vi "History.vi"() -> ()   [LabVIEW 2019]
uses:
  <vilib>/httpClient/LabVIEWHTTPClient.lvlib
  <vilib>/NI/AMC/AMC.lvlib
  <vilib>/addons/_JKI.lib/Serialization/JSON/JKI JSON Serialization.lvlib
  <vilib>/NI/Tools/String/Tools_String.lvlib
  <vilib>/Utility/miscctls.llb/LVPointTypeDef.ctl
  SCADA/Archive Viewer/TraceData.ctl
panel:
  in  "Data is log (value)":bool
  in  "seconds between data points (1 to 300 sec)":i32=10 min=1 max=300 step=1
  out "Calls to server":i32
  out "Num Points Returned":i32
  in  "Log Scale":bool
  out "XY Graph":cluster{timestamp[], dbl[]}[](graph)
  in  "Plot Data":bool
  in  "End Time":timestamp
  in  "Start Time":timestamp
  in  "Exit":bool
  in  "Select Traces":i32[](listbox)
  in  "Select Database":i32(listbox)
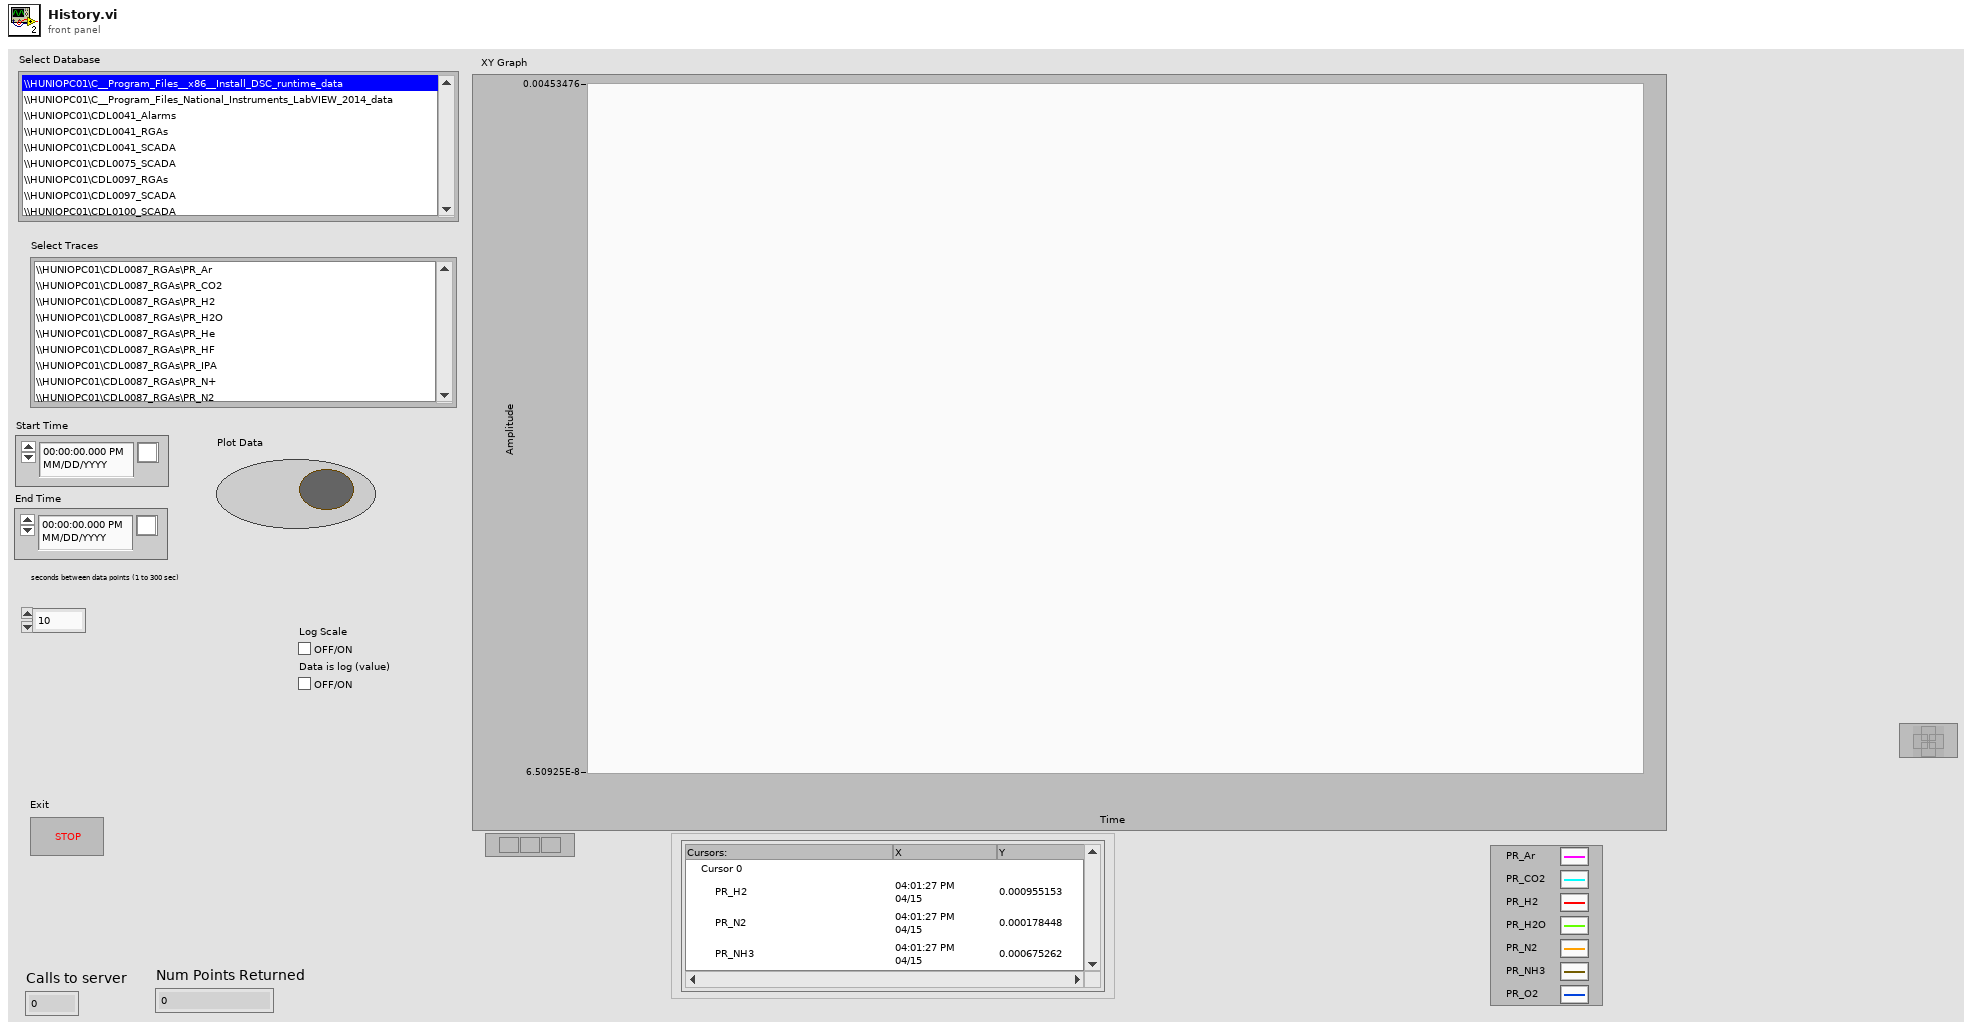
[diagram p1: front panel]
types:
  T1 = typedef "AMC.lvlib/Message Queue.ctl" = refnum<queue>
  T2 = typedef "LabVIEWHTTPClient.lvlib/ClientHandle.ctl" = refnum<k1>
  T3 = cluster{"firstTimestamp":string, "sampleInterval":i32, "data":dbl[]}
  T4 = typedef "LVPointTypeDef.ctl" = cluster{"Horizontal":i16, "Vertical":i16}
  T5 = typedef "TraceData.ctl" = cluster{"Trace":string, "LineWidth":u8, "TraceColor":u32, "DisplayName":string}
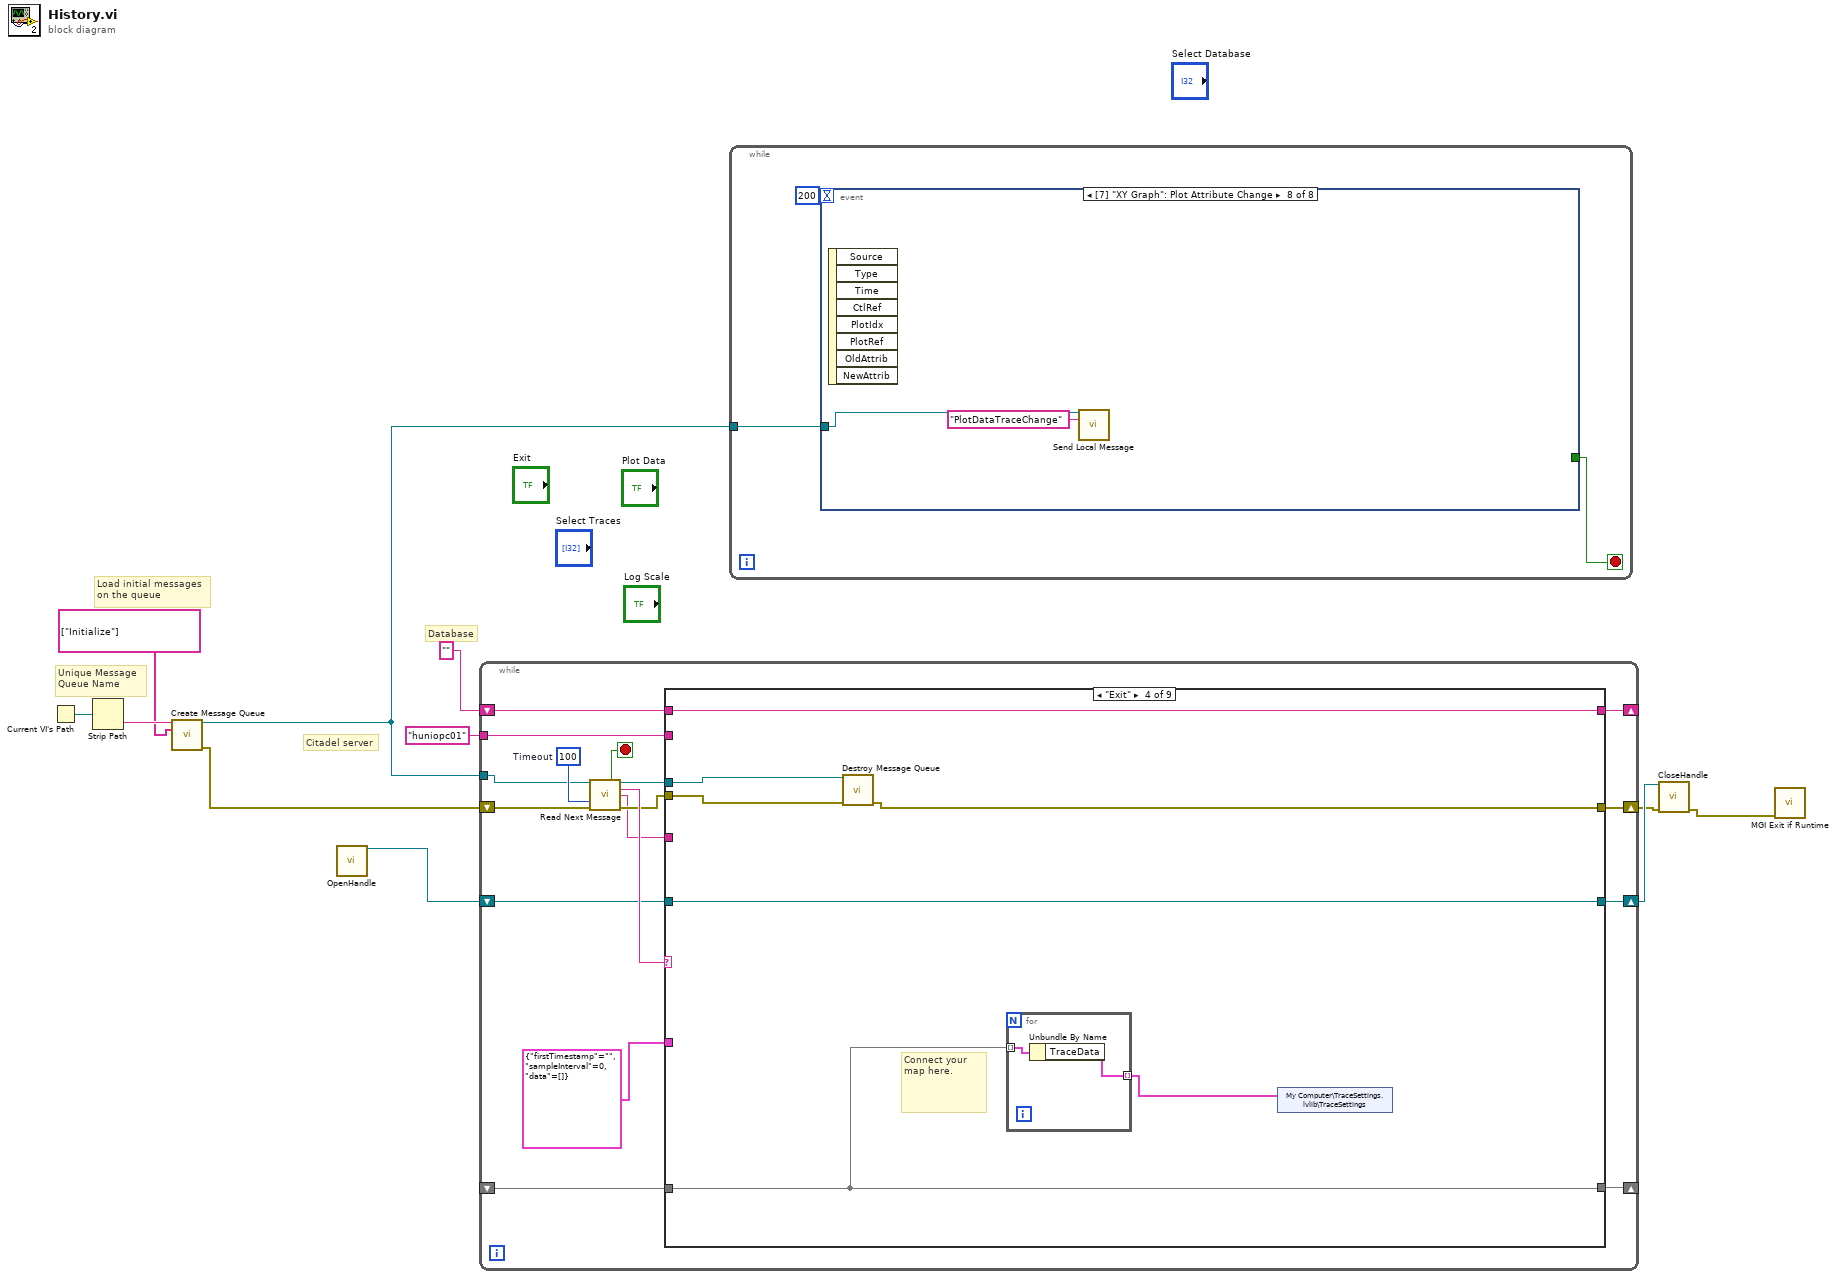
[diagram p0: block diagram]
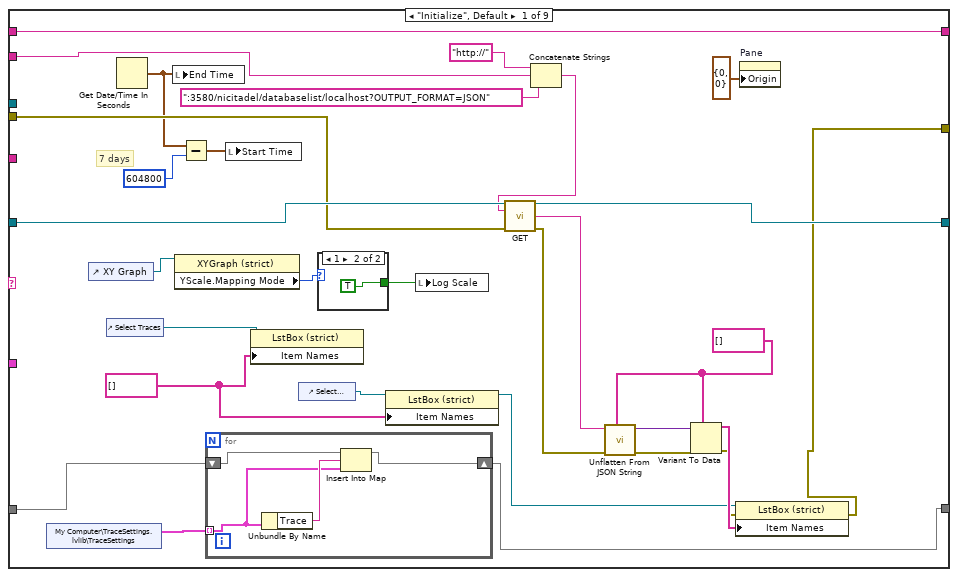
[diagram p2: hidden frame]
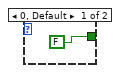
[diagram p3: hidden frame]
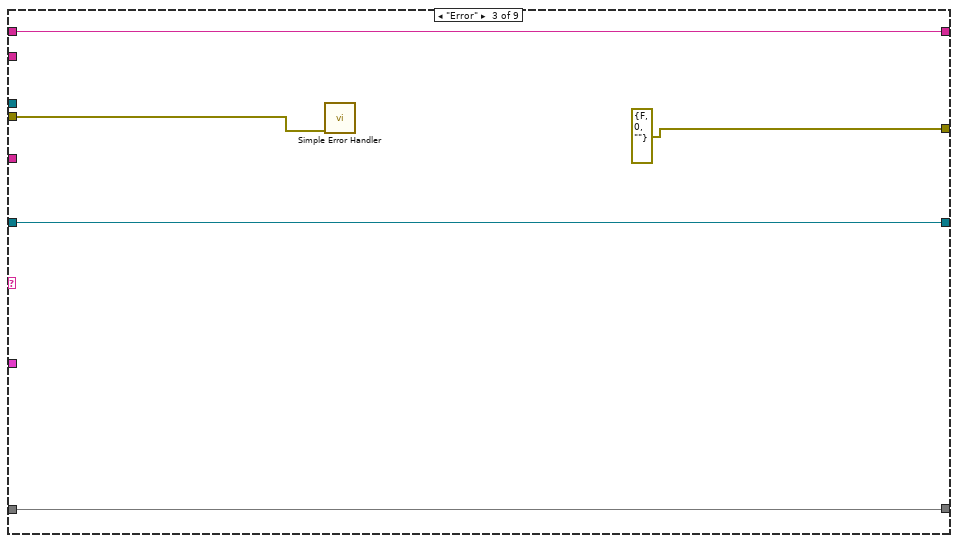
[diagram p5: hidden frame]
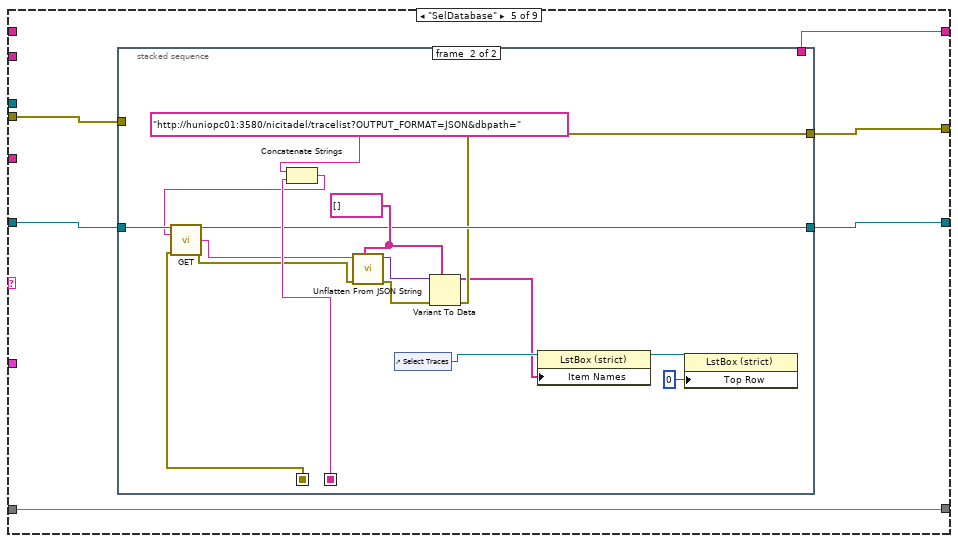
[diagram p6: hidden frame]
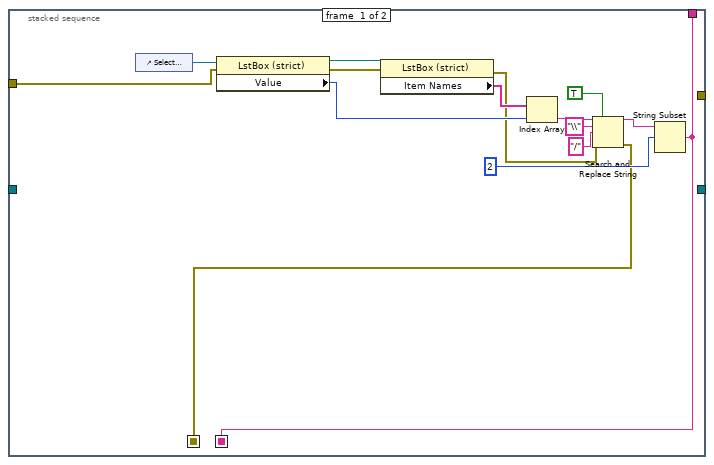
[diagram p7: hidden frame]
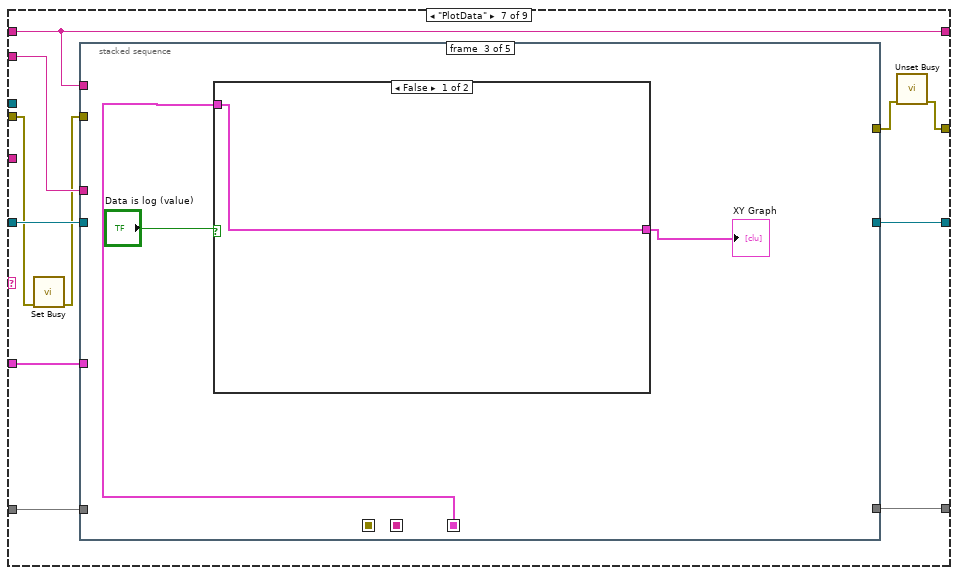
[diagram p9: hidden frame]
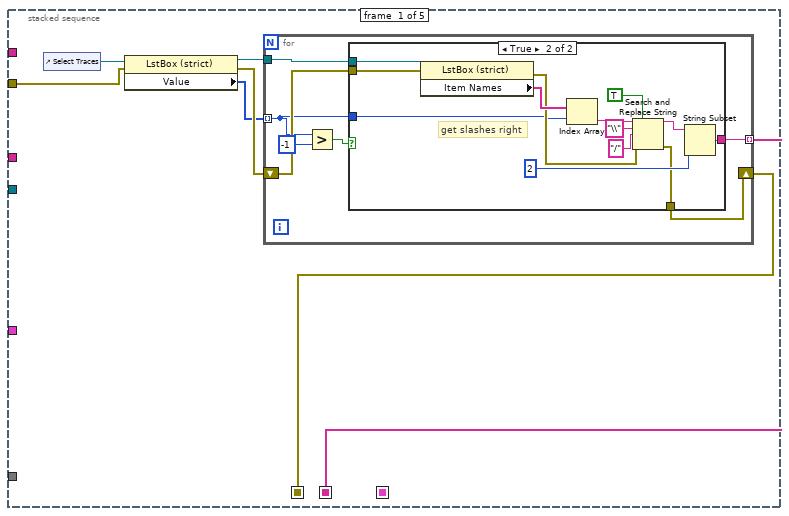
[diagram p10: hidden frame]
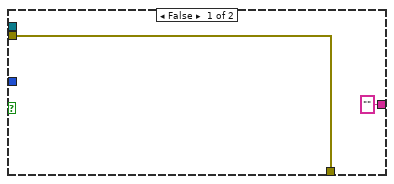
[diagram p11: hidden frame]
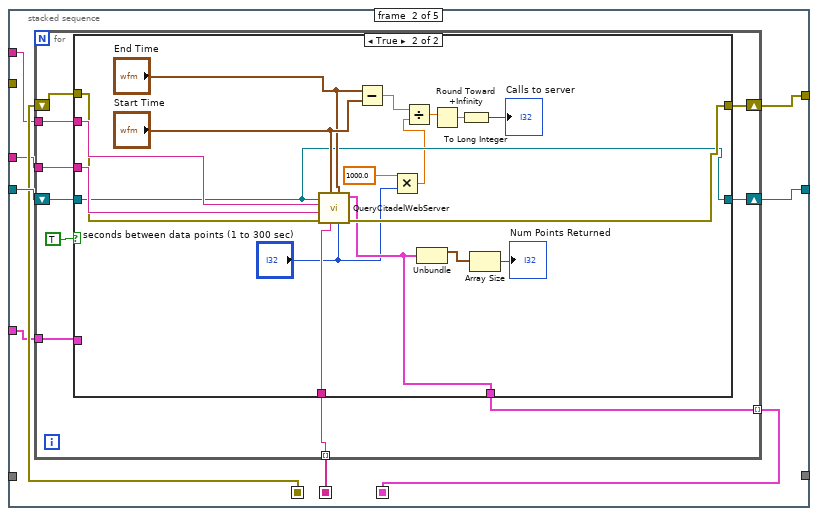
[diagram p12: hidden frame]
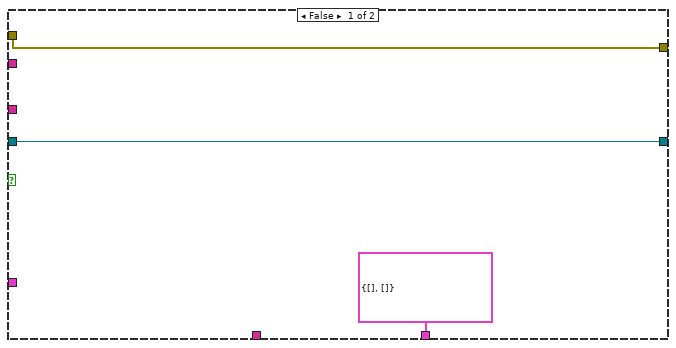
[diagram p13: hidden frame]
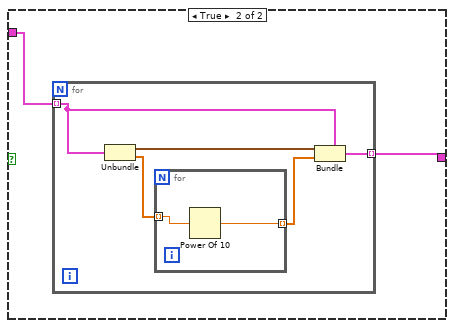
[diagram p14: hidden frame]
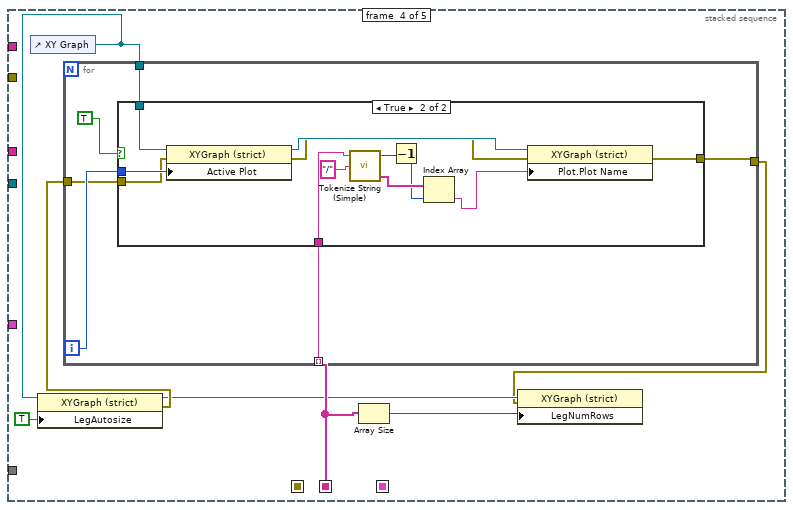
[diagram p15: hidden frame]
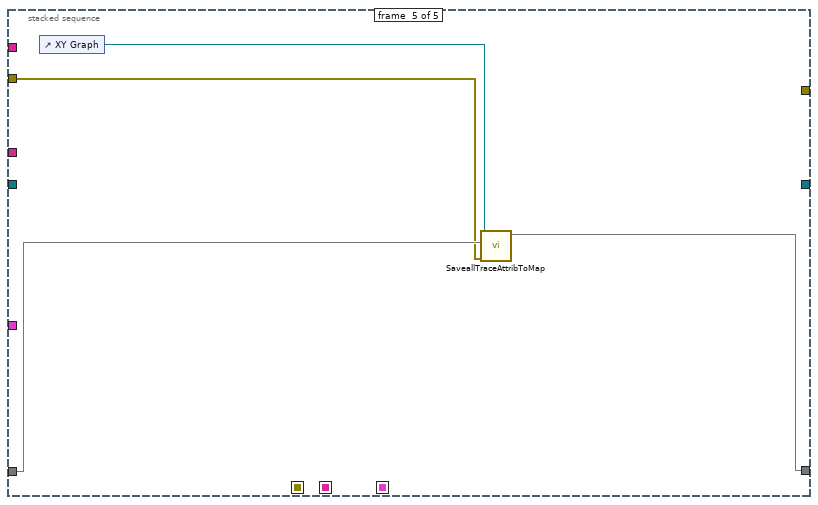
[diagram p17: hidden frame]
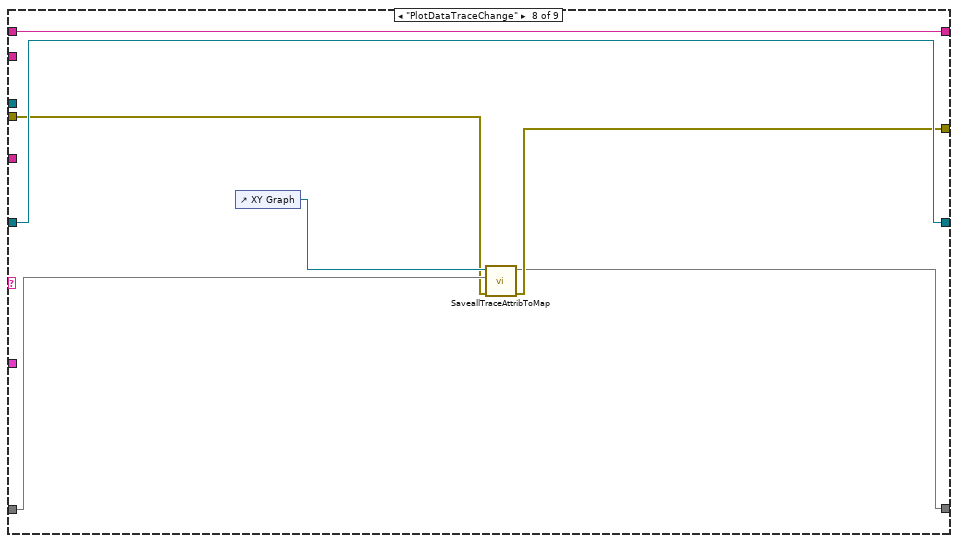
[diagram p18: hidden frame]
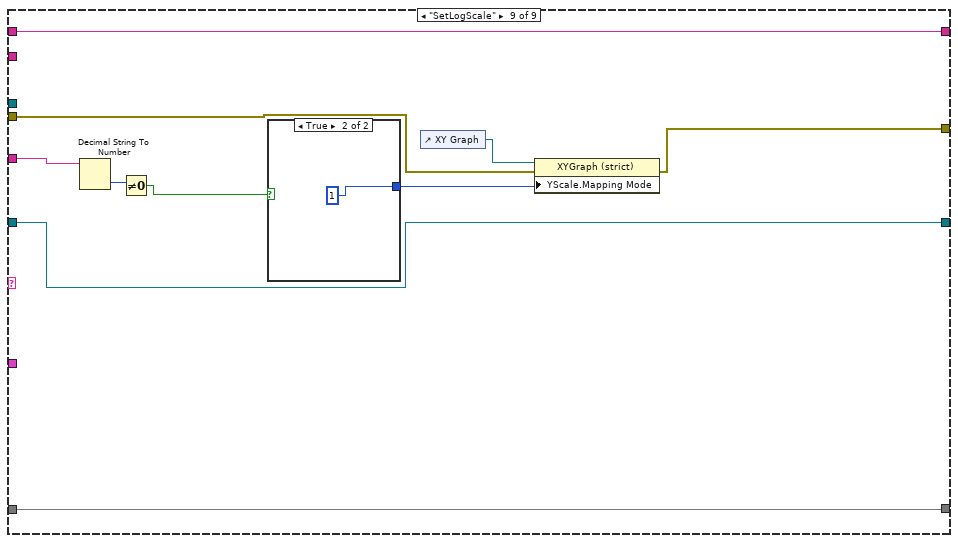
[diagram p19: hidden frame]
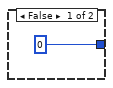
[diagram p20: hidden frame]
diagram:
  # "Database"
  # "Citadel server"
  # "Unique Message\nQueue Name"
  # "Load initial messages\non the queue"
  n1 = Current VI's Path() -> (path=w10:path)
  n2 = Strip Path(path=w10) -> (name=w11:string)  [unwired: 1 out]
  n3 = call <vilib>:"Create Message Queue.vi"("message queue name"=w11, "initial message names"=string[] ["Initialize"]) -> ("message queue out"=w4:T1, "error out"=w8:errorcluster)  [unwired: 12 in]
  n4 = call <vilib>:"OpenHandle.vi"() -> ("client handle out"=w7:T2)  [unwired: 14 in, 1 out]
  n5 = while {
    tunnel: w4 -> [w27]
    shift-right: [w20] -> w5
    shift-left: w8 -> [w26]
    shift-right: [w22] -> w6
    shift-left: w7 -> [w23]
    shift-right: [w17] -> _
    shift-left: "" -> [w18]
    tunnel: "huniopc01" -> [w15]
    shift-right: [w12] -> _
    shift-left: _ -> [w13]
    stop <- w25 stop-if-true
    w28 = 100  # Timeout
    n6 = call <vilib>:"Read Next Message.vi"("message queue in"=w27, "timeout (1 ms)"=w28, "error in"=w26) -> ("exit process?"=w25:bool, "message queue out"=w19:T1, "message name"=w24:string, "message value"=w14:string, "error out"=w21:errorcluster)  [unwired: 5 in, 3 out]
    n7 = case shown="\"Exit\"" w24 {
      tunnel: w23 -> [w55 w68 w71 w77 w87 w121 w134 w252 w258]
      tunnel: [w54 w68 w71 w77 w86 w121 w133 w252 w258] -> w22
      tunnel: w21 -> [w53 w67 w73 w79 w88 w122 w129 w249 w257]
      tunnel: [w48 w67 errorcluster {"status"=FALSE, "code"=0, "source"=""} ("error out") w78 w85 w122 w126 w248 w256] -> w20
      tunnel: w19 -> [_ _ _ w80 _ _ _ _ _]
      tunnel: w18 -> [w47 w66 w70 w76 _ w123 w132 w253 w255]
      tunnel: [w47 w66 w70 w76 w84 w123 w132 w253 w255] -> w17
      tunnel: T3 {"firstTimestamp"="", "sampleInterval"=0, "data"=[]} -> [_ _ _ _ _ _ w131 _ _]
      tunnel: w15 -> [w38 _ _ _ _ _ w130 _ _]
      tunnel: w14 -> [_ _ _ _ _ _ _ _ w263]
      tunnel: [w30 w65 w69 w75 w83 w120 w124 w247 w254] -> w12
      tunnel: w13 -> [w29 w65 w69 w75 w83 w120 w125 w250 w254]
      frame "Initialize", Default {
        w45 = string[] []
        w56 = string[] []
        # "7 days"
        n8 = shared-variable "My Computer\\TraceSettings.lvlib\\TraceSettings"() -> (w31:T5[])  [unwired: 1 in, 1 out]
        n9 = control-ref of="XY Graph"() -> (w35:refnum<vi>)
        n10 = control-ref of="Select Traces"() -> (w46:refnum<vi>)
        n11 = Get Date/Time In Seconds() -> (seconds since 1Jan1904=w42:timestamp)
        n12 = local write "End Time"(w42) -> ()
        n13 = property class="XYGraph (strict)"(reference=w35) -> ("YScale.Mapping Mode"=w34:u8)  [unwired: 1 in, 2 out]
        n14 = Subtract(x=w42, y=604800) -> (x-y=w40:timestamp)
        n15 = for {
          tunnel: w31 -> [w59] mode=indexing
          shift-right: [w61] -> w30
          shift-left: w29 -> [w62]
          n16 = Unbundle By Name(w59) -> ("Trace"=w60:string)
          n17 = Insert Into Map(map in=w62, key=w60, value=w59) -> (map out=w61:map{string, T5})  [unwired: 2 out]
        }
        n18 = local write "Start Time"(w40) -> ()
        n19 = property class="LstBox (strict)"(reference=w46, "Item Names"=w45) -> ()  [unwired: 1 in, 2 out]
        n20 = control-ref of="Select Database"() -> (w44:refnum<vi>)
        n21 = case shown="1" w34 {
          tunnel: [FALSE TRUE] -> w33
          frame 0, Default {
          }
          frame 1 {
          }
        }
        n22 = property class="LstBox (strict)"(reference=w44, "Item Names"=w45) -> (reference out=w43:refnum<vi>)  [unwired: 1 in, 1 out]
        n23 = local write "Log Scale"(w33) -> ()
        n24 = Concatenate Strings("http://" ("string"), w38, ":3580/nicitadel/databaselist/localhost?OUTPUT_FORMAT=JSON" ("url")) -> (w36:string)
        n25 = call <vilib>:"GET.vi"("client handle"=w55, "url"=w36, "error in (no error)"=w53) -> ("client handle out"=w54:T2, "body"=w58:string, "error out"=w52:errorcluster)  [unwired: 9 in, 1 out]
        n26 = call <vilib>:"Unflatten From JSON String.vi"("Type and Defaults"=w56, "error in (no error)"=w52, "JSON String"=w58) -> ("error out"=w51:errorcluster, "Variant"=w57:variant)  [unwired: 7 in]
        n27 = Variant To Data(error in=w51, type=w56, Variant=w57) -> (data=w50:string[], error out=w49:errorcluster)
        n28 = property class="LstBox (strict)"(reference=w43, error in=w49, "Item Names"=w50) -> (error out=w48:errorcluster)  [unwired: 1 out]
        n29 = property on="Pane" class="Pane"("Origin"=T4 {"Horizontal"=0, "Vertical"=0}) -> ()  [unwired: 2 in, 2 out]
      }
      frame "", "Idle" {
      }
      frame "Error" {
        n30 = call <vilib>:"Simple Error Handler.vi"("error in (no error)"=w73) -> ()  [unwired: 1 in, 8 out]
      }
      frame "Exit" {
        # "Connect your map here."
        n31 = call <vilib>:"Destroy Message Queue.vi"("message queue in"=w80, "error in"=w79) -> ("error out"=w78:errorcluster)  [unwired: 11 in, 2 out]
        n32 = for {
          tunnel: w75 -> [w82] mode=indexing
          tunnel: [w81] -> w74 mode=indexing
          n33 = Unbundle By Name(w82) -> ("TraceData"=w81:T5)
        }
        n34 = shared-variable "My Computer\\TraceSettings.lvlib\\TraceSettings"(w74) -> ()  [unwired: 1 in, 1 out]
      }
      frame "SelDatabase" {
        n35 = stacked-sequence {
          seq-local: [w90 _] -> [_ w118]
          seq-local: [w89 _] -> [_ w116]
          tunnel: w88 -> [w92 _]
          tunnel: w87 -> [_ w119]
          tunnel: [_ w109] -> w86
          tunnel: [_ w108] -> w85
          tunnel: [w89 _] -> w84
          frame #0 {
            n36 = control-ref of="Select Database"() -> (w97:refnum<vi>)
            n37 = property class="LstBox (strict)"(reference=w97, error in=w92) -> (reference out=w98:refnum<vi>, error out=w99:errorcluster, "Value"=w101:i32)
            n38 = property class="LstBox (strict)"(reference=w98, error in=w99) -> (error out=w91:errorcluster, "Item Names"=w100:string[])  [unwired: 1 out]
            n39 = Index Array(array=w100, index=w101) -> (element=w102:string)
            n40 = Search and Replace String(replace all?=TRUE ("replace all? (F)"), input string=w102, search string="\\", replace string="/" ("replace string (\"\")"), error in=w91) -> (result string=w103:string, error out=w90:errorcluster)  [unwired: 3 in, 2 out]
            n41 = String Subset(string=w103, offset (0)=2) -> (substring=w89:string)  [unwired: 1 in]
          }
          frame #1 {
            w112 = string[] []
            n42 = Concatenate Strings("http://huniopc01:3580/nicitadel/tracelist?OUTPUT_FORMAT=JSON&dbpath=" ("url"), w116) -> (w115:string)
            n43 = call <vilib>:"GET.vi"("client handle"=w119, "url"=w115, "error in (no error)"=w118) -> ("client handle out"=w109:T2, "body"=w114:string, "error out"=w110:errorcluster)  [unwired: 9 in, 1 out]
            n44 = call <vilib>:"Unflatten From JSON String.vi"("Type and Defaults"=w112, "error in (no error)"=w110, "JSON String"=w114) -> ("error out"=w111:errorcluster, "Variant"=w113:variant)  [unwired: 7 in]
            n45 = control-ref of="Select Traces"() -> (w107:refnum<vi>)
            n46 = Variant To Data(error in=w111, type=w112, Variant=w113) -> (data=w106:string[], error out=w108:errorcluster)
            n47 = property class="LstBox (strict)"(reference=w107, "Item Names"=w106) -> (reference out=w105:refnum<vi>)  [unwired: 1 in, 1 out]
            n48 = property class="LstBox (strict)"(reference=w105, "Top Row"=0) -> ()  [unwired: 1 in, 2 out]
          }
        }
      }
      frame "SelTrace" {
      }
      frame "PlotData" {
        n49 = call <vilib>:"Set Busy.vi"("error in (no error)"=w129) -> ("error out"=w128:errorcluster)  [unwired: 9 in, 1 out]
        n50 = stacked-sequence {
          seq-local: [w137 _ _ _ _] -> [_ w171 _ _ _]
          seq-local: [w136 _ _ _ _] -> [_ w170 _ w220 _]
          seq-local: [_ w164 _ _ _] -> [_ _ w206 _ _]
          tunnel: w128 -> [w138 _ _ _ w244]
          tunnel: w134 -> [_ w172 _ _ _]
          tunnel: [_ w169 _ _ _] -> w133
          tunnel: [_ w168 _ _ _] -> w127
          tunnel: w132 -> [_ w167 _ _ _]
          tunnel: w131 -> [_ w166 _ _ _]
          tunnel: w130 -> [_ w165 _ _ _]
          tunnel: w125 -> [_ _ _ _ w245]
          tunnel: [_ _ _ _ w243] -> w124
          frame #0 {
            n51 = control-ref of="Select Traces"() -> (w139:refnum<vi>)
            n52 = property class="LstBox (strict)"(reference=w139, error in=w138) -> (reference out=w140:refnum<vi>, error out=w141:errorcluster, "Value"=w135:i32[])
            n53 = for {
              tunnel: w140 -> [w147]
              tunnel: [w145] -> w136 mode=indexing
              tunnel: w135 -> [w142] mode=indexing
              shift-right: [w146] -> w137
              shift-left: w141 -> [w148]
              n54 = Greater?(x=w142, y=-1) -> (0:w143:bool)
              n55 = case shown="True" w143 {
                tunnel: w148 -> [w150 w160]
                tunnel: w147 -> [_ w159]
                tunnel: [w150 w153] -> w146
                tunnel: ["" ("result string") w152] -> w145
                tunnel: w142 -> [_ w151]
                frame False {
                }
                frame True {
                  # "get slashes right"
                  n56 = property class="LstBox (strict)"(reference=w159, error in=w160) -> (error out=w154:errorcluster, "Item Names"=w161:string[])  [unwired: 1 out]
                  n57 = Index Array(array=w161, index=w151) -> (element=w162:string)
                  n58 = Search and Replace String(replace all?=TRUE ("replace all? (F)"), input string=w162, search string="\\", replace string="/" ("replace string (\"\")"), error in=w154) -> (result string=w163:string, error out=w153:errorcluster)  [unwired: 3 in, 2 out]
                  n59 = String Subset(string=w163, offset (0)=2) -> (substring=w152:string)  [unwired: 1 in]
                }
              }
            }
          }
          frame #1 {
            n60 = for {
              tunnel: w170 -> [w180] mode=indexing
              tunnel: w167 -> [w177]
              tunnel: w165 -> [w174]
              shift-right: [w179] -> w169
              shift-left: w172 -> [w182]
              shift-right: [w178] -> w168
              shift-left: w171 -> [w181]
              tunnel: w166 -> [w176]
              tunnel: [w175] -> w164 mode=indexing
              n61 = case shown="True" TRUE {
                tunnel: w182 -> [w185 w192]
                tunnel: w181 -> [w184 w200]
                tunnel: w180 -> [_ w191]
                tunnel: [w185 w192] -> w179
                tunnel: [w184 w203] -> w178
                tunnel: w177 -> [_ w201]
                tunnel: w176 -> [_ _]
                tunnel: [cluster{timestamp[], dbl[]} {[], []} ("Data Out") w189] -> w175
                tunnel: w174 -> [_ w202]
                frame False {
                }
                frame True {
                  n62 = call <userlib>:"QueryCitadelWebServer.vi"("delta t data (s)"="seconds between data points (1 to 300 sec)", "End Time"="End Time", "Trace Names"=w191, "Start Time"="Start Time", "error in (no error)"=w200, "Server"=w202, "DB Path"=w201, "Refnum in"=w192) -> ("error out"=w203:errorcluster, "Data Out"=w189:cluster{timestamp[], dbl[]})  [unwired: 2 in]
                  n63 = Subtract(x="End Time", y="Start Time") -> (x-y=w197:dbl)
                  n64 = Multiply(x=1000.0 ("y"), y="seconds between data points (1 to 300 sec)") -> (x*y=w186:dbl)
                  n65 = Divide(x=w197, y=w186) -> (x/y=w196:dbl)
                  n66 = Unbundle(w189) -> (w190:timestamp[])  [unwired: 1 out]
                  n67 = Round Toward +Infinity(x=w196) -> (ceil(x): smallest int >= x=w195:dbl)
                  n68 = To Long Integer(number=w195) -> (32bit integer=→"Calls to server":i32)
                  n69 = Array Size(array=w190) -> (size(s)=→"Num Points Returned":i32)
                }
              }
            }
          }
          frame #2 {
            n70 = case shown="False" "Data is log (value)" {
              tunnel: w206 -> [w207 w209]
              tunnel: [w207 w208] -> w204
              frame False {
              }
              frame True {
                n71 = for {
                  tunnel: w209 -> [w213] mode=indexing
                  tunnel: [w210] -> w208 mode=indexing
                  n72 = Unbundle(w213) -> (w212:timestamp[], w214:dbl[])
                  n73 = for {
                    tunnel: w214 -> [w216] mode=indexing
                    tunnel: [w215] -> w211 mode=indexing
                    n74 = Power Of 10(x=w216) -> (10^x=w215:dbl)
                  }
                  n75 = Bundle(cluster=w213, w212, w211) -> (w210:cluster{timestamp[], dbl[]})
                }
              }
            }
            "XY Graph" <- w204
          }
          frame #3 {
            n76 = control-ref of="XY Graph"() -> (w223:refnum<vi>)
            n77 = property class="XYGraph (strict)"(reference=w223, "LegAutosize"=TRUE ("Legend:Autosize")) -> (reference out=w219:refnum<vi>, error out=w222:errorcluster)  [unwired: 1 in]
            n78 = for {
              tunnel: w220 -> [w229] mode=indexing
              tunnel: w223 -> [w227]
              tunnel: w222 -> [w225]
              tunnel: [w224] -> w218
              i -> [w226]
              n79 = case shown="True" TRUE {
                tunnel: w229 -> [_ w242]
                tunnel: w227 -> [_ w236]
                tunnel: w226 -> [_ w234]
                tunnel: w225 -> [w230 w232]
                tunnel: [w230 w231] -> w224
                frame False {
                }
                frame True {
                  n80 = property class="XYGraph (strict)"(reference=w236, error in=w232, "Active Plot"=w234) -> (reference out=w235:refnum<vi>, error out=w233:errorcluster)
                  n81 = call <vilib>:"Tokenize String (Simple).vi"("delimiter ([\\s\\t\\n\\r]+)"="/" ("delimiter ([\\s\\t\\n\\r]+)"), "input string"=w242) -> ("token array"=w240:string[], "number of tokens"=w239:i32)  [unwired: 2 in]
                  n82 = Decrement(x=w239) -> (x-1=w238:i32)
                  n83 = Index Array(array=w240, index=w238) -> (element=w237:string)
                  n84 = property class="XYGraph (strict)"(reference=w235, error in=w233, "Plot.Plot Name"=w237) -> (error out=w231:errorcluster)  [unwired: 1 out]
                }
              }
            }
            n85 = Array Size(array=w220) -> (size(s)=w217:i32)
            n86 = property class="XYGraph (strict)"(reference=w219, error in=w218, "LegNumRows"=w217) -> ()  [unwired: 2 out]
          }
          frame #4 {
            n87 = control-ref of="XY Graph"() -> (w246:refnum<vi>)
            n88 = call "SaveallTraceAttribToMap.vi"("error in (no error)"=w244, "Map in"=w245, "XYGraph in"=w246) -> ("Map out"=w243:map{string, T5})  [unwired: 7 in, 1 out]
          }
        }
        n89 = call <vilib>:"Unset Busy.vi"("error in (no error)"=w127) -> ("error out"=w126:errorcluster)  [unwired: 10 in]
      }
      frame "PlotDataTraceChange" {
        n90 = control-ref of="XY Graph"() -> (w251:refnum<vi>)
        n91 = call "SaveallTraceAttribToMap.vi"("error in (no error)"=w249, "Map in"=w250, "XYGraph in"=w251) -> ("error out"=w248:errorcluster, "Map out"=w247:map{string, T5})  [unwired: 7 in]
      }
      frame "SetLogScale" {
        n92 = Decimal String To Number(string=w263) -> (number=w262:i32)  [unwired: 2 in, 1 out]
        n93 = Not Equal To 0?(x=w262) -> (x != 0?=w261:bool)
        n94 = case shown="True" w261 {
          tunnel: [u8 0 ("Y Scale.Mapping Mode") u8 1 ("Y Scale.Mapping Mode")] -> w259
          frame False {
          }
          frame True {
          }
        }
        n95 = control-ref of="XY Graph"() -> (w260:refnum<vi>)
        n96 = property class="XYGraph (strict)"(reference=w260, error in=w257, "YScale.Mapping Mode"=w259) -> (error out=w256:errorcluster)  [unwired: 1 out]
      }
    }
  }
  n97 = while {
    tunnel: w4 -> [w266]
    stop <- w267 stop-if-true
    n98 = event shown="[7] \"XY Graph\": Plot Attribute Change" {
      selector: _ -> [_ _ _ _ _ _ _ _]
      dyn-events: _ -> [_ _ _ _ _ _ _ _]
      timeout: 200 -> [_ _ _ _ _ _ _ _]
      tunnel: [w269 _ w275 _ _ _ _ _] -> w267
      tunnel: w266 -> [w271 w272 w276 w280 w282 w287 w289 w293]
      event Timeout {
        n99 = event-data() -> ()  [unwired: 1 in, 3 out]
        n100 = call <vilib>:"Check Message Queue Status.vi"("message queue in"=w271) -> ("error out"=w270:errorcluster)  [unwired: 10 in, 4 out]
        n101 = Unbundle By Name(w270) -> ("status"=w269:bool)
      }
      event Panel Close? {
        n102 = event-data() -> ()  [unwired: 1 in, 4 out]
        n103 = call <vilib>:"Send Local Message.vi"("message queue in"=w272, "message name"="Exit") -> ()  [unwired: 11 in, 3 out]
        n104 = event-data("Discard?"=TRUE) -> ()  [unwired: 1 in, 1 out]
      }
      event "Exit": Value Change {
        n105 = event-data() -> ("NewVal"=w275:bool)  [unwired: 1 in, 5 out]
        n106 = case shown="True" w275 {
          tunnel: w276 -> [_ w277]
          frame False {
          }
          frame True {
            n107 = call <vilib>:"Send Local Message.vi"("message queue in"=w277, "message name"="Exit") -> ()  [unwired: 11 in, 3 out]
          }
        }
      }
      event "Select Database": Value Change {
        n108 = event-data() -> ()  [unwired: 1 in, 6 out]
        n109 = call <vilib>:"Send Local Message.vi"("message queue in"=w280, "message name"="SelDatabase") -> ()  [unwired: 11 in, 3 out]
      }
      event "Select Traces": Value Change {
        n110 = event-data() -> ()  [unwired: 1 in, 6 out]
        n111 = call <vilib>:"Send Local Message.vi"("message queue in"=w282, "message name"="SelTrace") -> ()  [unwired: 11 in, 3 out]
      }
      event "Log Scale": Value Change {
        n112 = event-data() -> ("NewVal"=w285:bool)  [unwired: 1 in, 5 out]
        n113 = Boolean To (0,1)(Boolean=w285) -> (0, 1=w284:i16)
        n114 = Number To Decimal String(number=w284) -> (decimal integer string=w283:string)  [unwired: 1 in]
        n115 = call <vilib>:"Send Local Message.vi"("message queue in"=w287, "message name"="SetLogScale", "message value"=w283) -> ()  [unwired: 10 in, 3 out]
      }
      event "Plot Data": Value Change {
        n116 = event-data() -> ("NewVal"=w288:bool)  [unwired: 1 in, 5 out]
        n117 = case shown="True" w288 {
          tunnel: w289 -> [_ w291]
          frame False {
          }
          frame True {
            n118 = call <vilib>:"Send Local Message.vi"("message queue in"=w291, "message name"="PlotData") -> ()  [unwired: 11 in, 3 out]
          }
        }
      }
      event "XY Graph": Plot Attribute Change {
        n119 = event-data() -> ()  [unwired: 1 in, 8 out]
        n120 = call <vilib>:"Send Local Message.vi"("message queue in"=w293, "message name"="PlotDataTraceChange") -> ()  [unwired: 11 in, 3 out]
      }
    }
  }
  n121 = call <vilib>:"CloseHandle.vi"("client handle"=w6, "error in (no error)"=w5) -> ("error out"=w1:errorcluster)  [unwired: 13 in]
  n122 = call <userlib>:"MGI Exit if Runtime.vi"("Error In (Dependency Only)"=w1) -> ()  [unwired: 11 in]
